vi "WSVCAP SHL Host TL RFFE Read - Multiple DUTs - Common Data.vi"(0 "Data Out":string, 11 "error in":errorcluster, 13 "DUT Mask (All)":bool[](array[boolean])=[TRUE, TRUE, TRUE, TRUE, TRUE, TRUE, TRUE, TRUE, TRUE, TRUE, TRUE, TRUE, TRUE, TRUE, TRUE, TRUE]) -> (4 "RFFE Data In":string[](array[string]), 15 "error out":errorcluster)   [LabVIEW 2012]
panel:
  out "RFFE Data In [U8]":u8[][](array[numeric]) format="%02x"
  out "Socket Mask":u16=1 format="%02x"
  # "DUT 01"
  # "DUT 02"
  # "DUT 03"
  # "DUT 04"
  # "DUT 05"
  # "DUT 06"
  # "DUT 07"
  # "DUT 08"
  # "DUT 09"
  # "DUT 10"
  # "DUT 11"
  # "DUT 12"
  # "DUT 13"
  # "DUT 14"
  # "DUT 15"
  # "DUT 16"
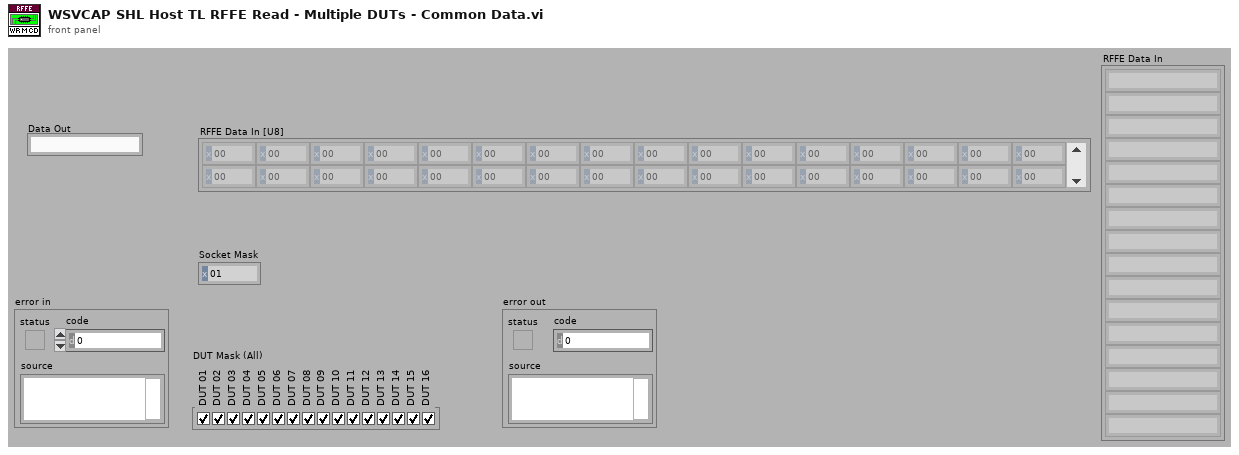
[diagram p1: front panel]
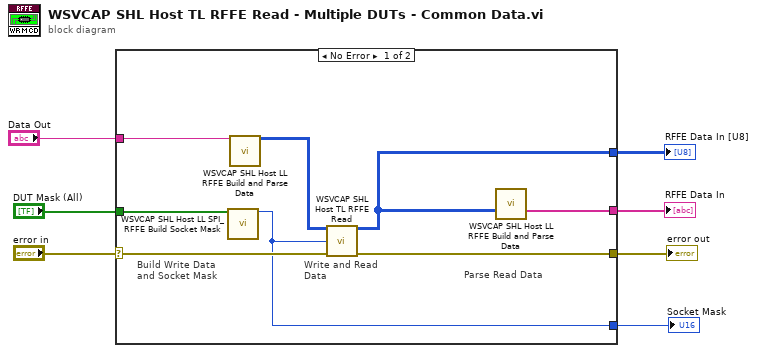
[diagram p0: block diagram]
diagram:
  n1 = case shown="No Error" "error in" {
    selector: "error in" -> [w14 _]
    tunnel: [w15 _] -> w7
    tunnel: [w10 _] -> w5
    tunnel: "DUT Mask (All)" -> [w13 _]
    tunnel: [w12 _] -> w3
    tunnel: [w11 _] -> w2
    tunnel: "Data Out" -> [w9 _]
    frame No Error {
      # "Parse Read Data"
      # "Write and Read\nData"
      # "Build Write Data and Socket Mask"
      n2 = call "WSVCAP SHL Host LL SPI_RFFE Build Socket Mask.vi"("DUT Mask"=w13) -> ("Socket Mask [U16]"=w10:u16)  [unwired: 13 in, 1 out]
      n3 = call "WSVCAP SHL Host LL RFFE Build and Parse Data.vi"("Data Out"=w9) -> ("RFFE Data Out [U8]"=w8:u8[][])  [unwired: 11 in, 3 out]
      n4 = call "WSVCAP SHL Host TL RFFE Read.vi"("Write Data In [DUT Ordered]"=w8, "Socket Mask"=w10, "error in"=w14) -> ("Read Data Out"=w12:u8[][], "error out"=w15:errorcluster)  [unwired: 11 in]
      n5 = call "WSVCAP SHL Host LL RFFE Build and Parse Data.vi"("RFFE Data In [U8]"=w12) -> ("RFFE Data In"=w11:string[])  [unwired: 11 in, 3 out]
    }
    frame Error {
    }
  }
  "error out" <- w7
  "Socket Mask" <- w5
  "RFFE Data In" <- w2
  "RFFE Data In [U8]" <- w3
